vi "Update Engine Stream Filter.vi"(8 "error in (no error)":errorcluster, 10 "Filter":T1, 11 "Refs":T4 {"Termination" items=["Off", "On"]}) -> (0 "error out":errorcluster)   [LabVIEW 2019, in "CAN Streaming Support Engine.lvlib"]
uses:
  CAN Streaming Support Engine.lvlib
  Types/Engine Stream API Refs.ctl
  Addon Shared/Types/Direction Filter.ctl
  Addon Shared/Types/Type Filter.ctl
  Addon Shared/Types/Filter Parameters.ctl
  Addon Shared/CAN Streaming Support Shared.lvlib
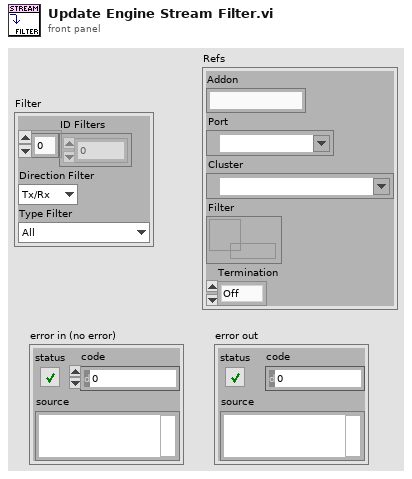
[diagram p1: front panel]
types:
  T1 = typedef "CAN Streaming Support Shared.lvlib/Filter Parameters.ctl" = cluster{"ID Filters":u32[], "Direction Filter":T2, "Type Filter":T3}
  T2 = typedef "CAN Streaming Support Shared.lvlib/Direction Filter.ctl" = enum16{"Tx/Rx", "Rx", "Tx"}
  T3 = typedef "CAN Streaming Support Shared.lvlib/Type Filter.ctl" = enum16{"All", "CAN Data", "CAN Remote", "CAN Bus Error", "CAN 2.0 Data", "CAN FD Data", "CAN FD+BRS Data", "J1939 Data", "Delay", "Log Trigger", "Start Trigger"}
  T4 = typedef "CAN Streaming Support Engine.lvlib/Engine Stream API Refs.ctl" = cluster{"Addon":string, "Port":refnum<k21>, "Cluster":refnum<k21>, "Filter":refnum<data-value>, "Termination":u32}
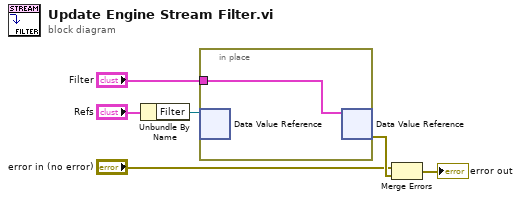
[diagram p0: block diagram]
diagram:
  n1 = Unbundle By Name("Refs") -> ("Filter"=w2:refnum<data-value>)
  n2 = in-place {
    in-place-border: "Filter" -> [w7]
    n3 = in-place-dvr #1(w2) -> ()  [unwired: 2 out]
    n4 = in-place-dvr #1(w7) -> (w5:errorcluster)  [unwired: 1 out]
  }
  n5 = Merge Errors("error in (no error)", w5) -> (→"error out":errorcluster)
